vi "pidtry.vi"() -> ()   [LabVIEW 2015]
uses:
  <vilib>/DAQmx/write.llb/DAQmx Write (Analog DBL 1Chan 1Samp).vi
  <vilib>/DAQmx/read.llb/DAQmx Read (Analog DBL 1Chan 1Samp).vi
  <vilib>/DAQmx/create/channels.llb/DAQmx Create Channel (AI-Voltage-Basic).vi
  <vilib>/DAQmx/configure/timing.llb/DAQmx Timing (Sample Clock).vi
  <vilib>/DAQmx/create/channels.llb/DAQmx Create Channel (AO-Voltage-Basic).vi
  <vilib>/DAQmx/miscellaneous.llb/DAQmx Fill In Error Info.vi
panel:
  in  "Blink Speed (CH1) 2":dbl min=0.0 max=3.3 step=0.1
  in  "Motor Speed (CH1)":dbl min=0.0 max=3.3 step=0.1
  out "Waveform Chart":dbl(graph)
  in  "stop":bool
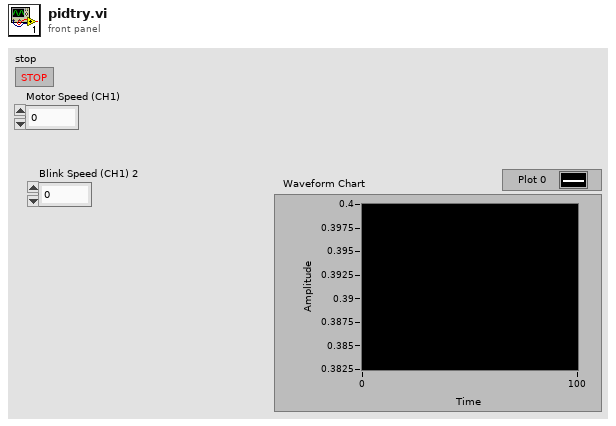
[diagram p1: front panel]
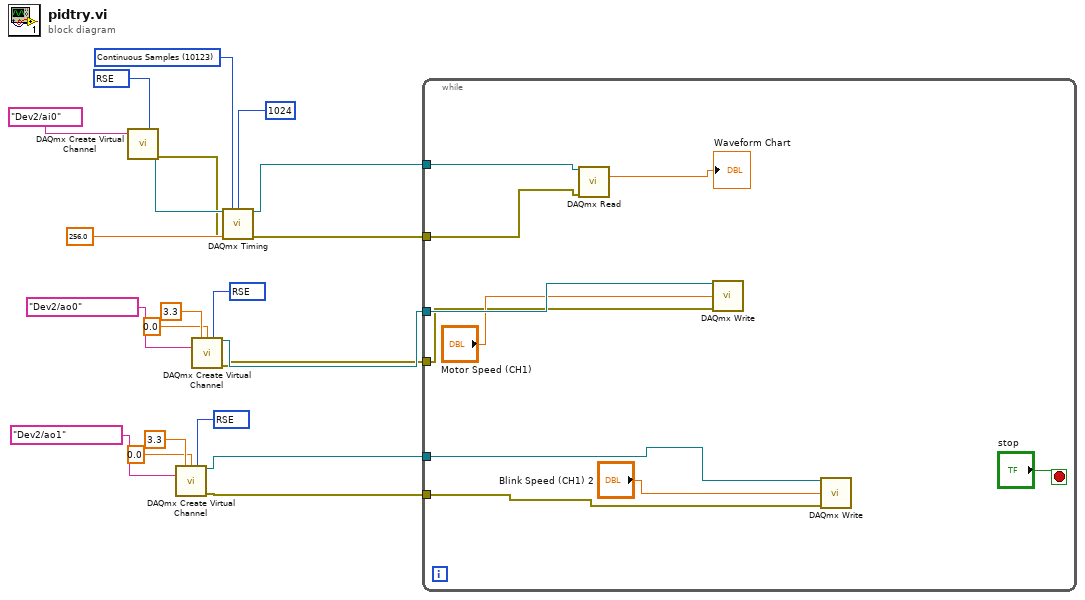
[diagram p0: block diagram]
diagram:
  w8 = 10083 items=["Default"=-1, "RSE"=10083, "Differential"=10106, "Pseudodifferential"=12529] ("output terminal configuration")
  w14 = 10083 items=["Default"=-1, "RSE"=10083, "NRSE"=10078, "Differential"=10106, "Pseudodifferential"=12529] ("input terminal configuration")
  w15 = 10083 items=["Default"=-1, "RSE"=10083, "Differential"=10106, "Pseudodifferential"=12529] ("output terminal configuration")
  w19 = 10123 items=["Finite Samples"=10178, "Continuous Samples"=10123, "Hardware Timed Single Point"=12522] ("sample mode")
  n1 = call-poly <vilib>:"DAQmx Create Virtual Channel.vi"("input terminal configuration"=w14, "physical channels"=tag "Dev2/ai0") -> ("task out"=w20:refnum<k21>, "error out"=w13:errorcluster)  [unwired: 12 in]
  n2 = call-poly <vilib>:"DAQmx Create Virtual Channel.vi"("maximum value"=3.3, "minimum value"=0.0, "output terminal configuration"=w8, "physical channels"=tag "Dev2/ao1") -> ("task out"=w6:refnum<k21>, "error out"=w5:errorcluster)  [unwired: 10 in]
  n3 = call-poly <vilib>:"DAQmx Create Virtual Channel.vi"("maximum value"=3.3, "minimum value"=0.0, "output terminal configuration"=w15, "physical channels"=tag "Dev2/ao0") -> ("task out"=w10:refnum<k21>, "error out"=w9:errorcluster)  [unwired: 10 in]
  n4 = call-poly <vilib>:"DAQmx Timing.vi"("task/channels in"=w20, "sample mode"=w19, "samples per channel"=1024, "rate"=256.0, "error in"=w13) -> ("task out"=w17:refnum<k21>, "error out"=w16:errorcluster)  [unwired: 9 in]
  n5 = while {
    tunnel: w17 -> [w30]
    tunnel: w16 -> [w29]
    tunnel: w10 -> [w27]
    tunnel: w9 -> [w25]
    tunnel: w6 -> [w23]
    tunnel: w5 -> [w22]
    stop <- "stop" stop-if-true
    n6 = call-poly <vilib>:"DAQmx Read.vi"("task/channels in"=w30, "error in"=w29) -> ("data"=→"Waveform Chart":dbl)  [unwired: 11 in, 2 out]
    n7 = call-poly <vilib>:"DAQmx Write.vi"("task/channels in"=w27, "data"="Motor Speed (CH1)", "error in"=w25) -> ()  [unwired: 10 in, 3 out]
    n8 = call-poly <vilib>:"DAQmx Write.vi"("task/channels in"=w23, "data"="Blink Speed (CH1) 2", "error in"=w22) -> ()  [unwired: 10 in, 3 out]
  }
